vi "ISEG_HVChannel.destructor.vi"(0 "i ref in":refnum<vi>, 5 "error in (no error)":errorcluster) -> (19 "error out":errorcluster)   [LabVIEW 2014, in "ISEG_HVChannel.lvlib"]
doc: "This is the destructor of a class.\n\nLicense Agreement for this software:\n\nCopyright (C)\nGesellschaft für Schwerionenforschung, GSI\nPlanckstr. 1\n64291 Darmstadt\nGermany\n\nContact: D.Beck@gsi.de \n\nThis program is free software; you can redistribute it and/or modify it under the terms of the \nGNU General Public License as published by the Free Software Foundation; either version 2 of \nthe license, or (at your option) any later version.\n\nThis program is distributed in the hope that it will be useful, but WITHOUT ANY WARRANTY; \nwithout even the implied warranty of MERCHANTABILITY or FITNESS FOR A PARTICULAR PURPOSE. See the GNU General License for more details (http://www.gnu.org).\n\nGesellschaft für Schwerionenforschung, GSI\nPlanckstr. 1, 64291 Darmstadt, Germany\nFor all questions and ideas contact: M.Richter@gsi.de, H.Brand@gsi.de or D.Beck@gsi.de.\nLast update: 16-JUN-2004"
uses:
  ISEG_HVChannel.lvlib
  CS_Core/CSApplicationBaseClasses/PSChannelBase/PSChannelBase.lvlib
  CSlibraries-extern/DimLVEvent/LVDimInterface/LVDimInterface.lvlib
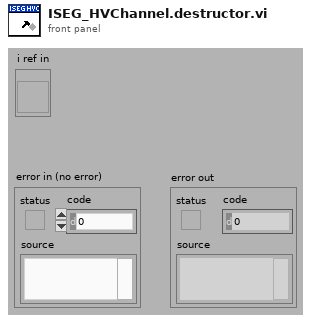
[diagram p1: front panel]
types:
  T1 = typedef "ISEG_HVChannel.lvlib/ISEG_HVChannel.i attribute.ctl" = cluster{"Channel Array":cluster{"Logical Name":string, "Address":string, "error in (no error)":errorcluster, "Status":cluster{"Status":i16, "DIM Status":T2}, "On":cluster{"On":bool, "DIM Status":T2}, "VMeas ":cluster{"VMeas":dbl, "DIM Status":T2}, "VSet ":cluster{"VSet":dbl, "DIM Status":T2}, "ITrip ":cluster{"ITrip":dbl, "DIM Status":T2}, "IMeas":cluster{"IMeas":dbl, "DIM Status":T2}, " RampSpeed":cluster{"RampSpeed":dbl, "DIM Status":T2}, "EventMask ":cluster{"EventMask":i16, "DIM Status":T2}}[], "VoltageInRangeBand":dbl, "NofCh":cluster{"NofCh":i32, "DIM Service":i32}, "BoardPrefix":string}
  T2 = typedef "ISEG_HVChannel.lvlib/ISEG_HVChannel.DIM Status.ctl" = cluster{"no link":bool, "quality":i32, "Time Stamp":timestamp}
  T3 = enum16{"SetAttribute", "GetAttribute", "CreateAttribute", "DestroyAttribute", "DestroyAllAtributes"}
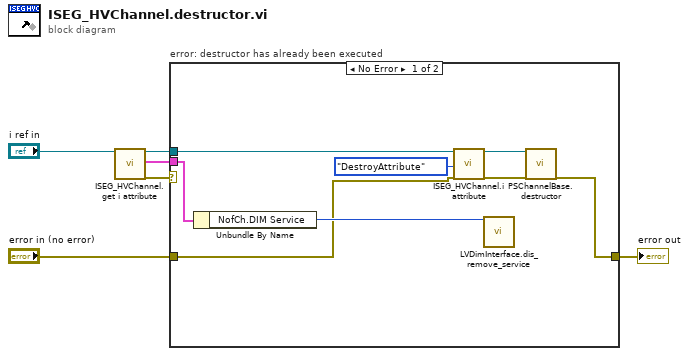
[diagram p0: block diagram]
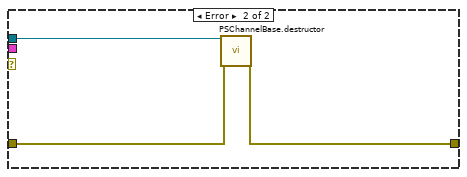
[diagram p2: hidden frame]
diagram:
  n1 = call "ISEG_HVChannel.get i attribute.vi"("i ref in"="i ref in") -> ("i ref out"=w2:refnum<vi>, "i attribute"=w1:T1, "error out"=w3:errorcluster)  [unwired: 16 in]
  n2 = case "error: destructor has already been executed" shown="No Error" w3 {
    tunnel: [w11 w15] -> w6
    tunnel: "error in (no error)" -> [w7 w16]
    tunnel: w2 -> [w8 w17]
    tunnel: w1 -> [w10 _]
    frame No Error {
      n3 = Unbundle By Name(w10) -> ("NofCh.DIM Service"=w9:i32)
      n4 = call "ISEG_HVChannel.i attribute.vi"("VI Refnum"=w8, "Action"=T3."DestroyAttribute", "error in (no error)"=w7) -> ("VI Refnum out"=w13:refnum<vi>, "error out"=w12:errorcluster)  [unwired: 14 in, 1 out]
      n5 = call "LVDimInterface.dis_remove_service.vi"("my_serviceID"=w9) -> ()  [unwired: 18 in, 1 out]
      n6 = call "PSChannelBase.destructor.vi"("i ref in"=w13, "error in (no error)"=w12) -> ("error out"=w11:errorcluster)  [unwired: 17 in]
    }
    frame Error {
      n7 = call "PSChannelBase.destructor.vi"("i ref in"=w17, "error in (no error)"=w16) -> ("error out"=w15:errorcluster)  [unwired: 17 in]
    }
  }
  "error out" <- w6
